vi "sub_LidarTrimPlot.vi"(0 "R_min":dbl=0.3 format="%#_13g", 1 "UDP 네트워크 연결 입력":refnum<k16>, 5 "x-":dbl=-1.0, 7 "x+":dbl=1.0, 9 "y-":dbl, 11 "y+":dbl=8.0, 12 "에러 입력(에러 없음)":errorcluster) -> (3 "UDP 네트워크 연결 출력":refnum<k16>, 4 "Point Cloud Plotting":cluster{"X":dbl, "Y":dbl}[](graph), 6 "trim XY DATA":cluster{"X":dbl, "Y":dbl}[](array[cluster]), 14 "에러 출력":errorcluster)   [LabVIEW 2020]
panel:
  in  "탭 컨트롤":enum32{"인디케이터"}(tab)
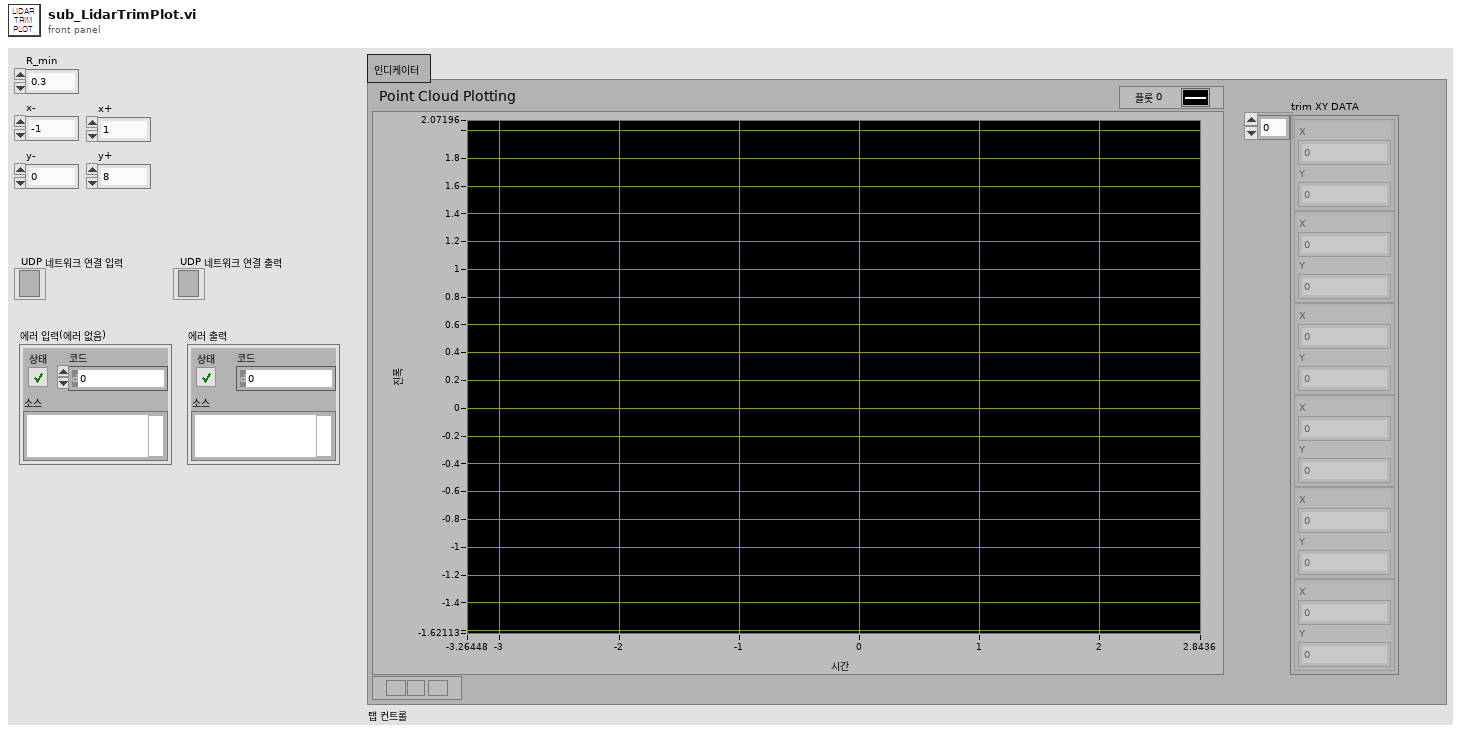
[diagram p1: front panel]
types:
  T1 = cluster{"id":i32, "azimuth (degree)":dbl, "vertical (degree)":dbl, "distance (meter)":dbl, "X":dbl, "Y":dbl, "Z":dbl}
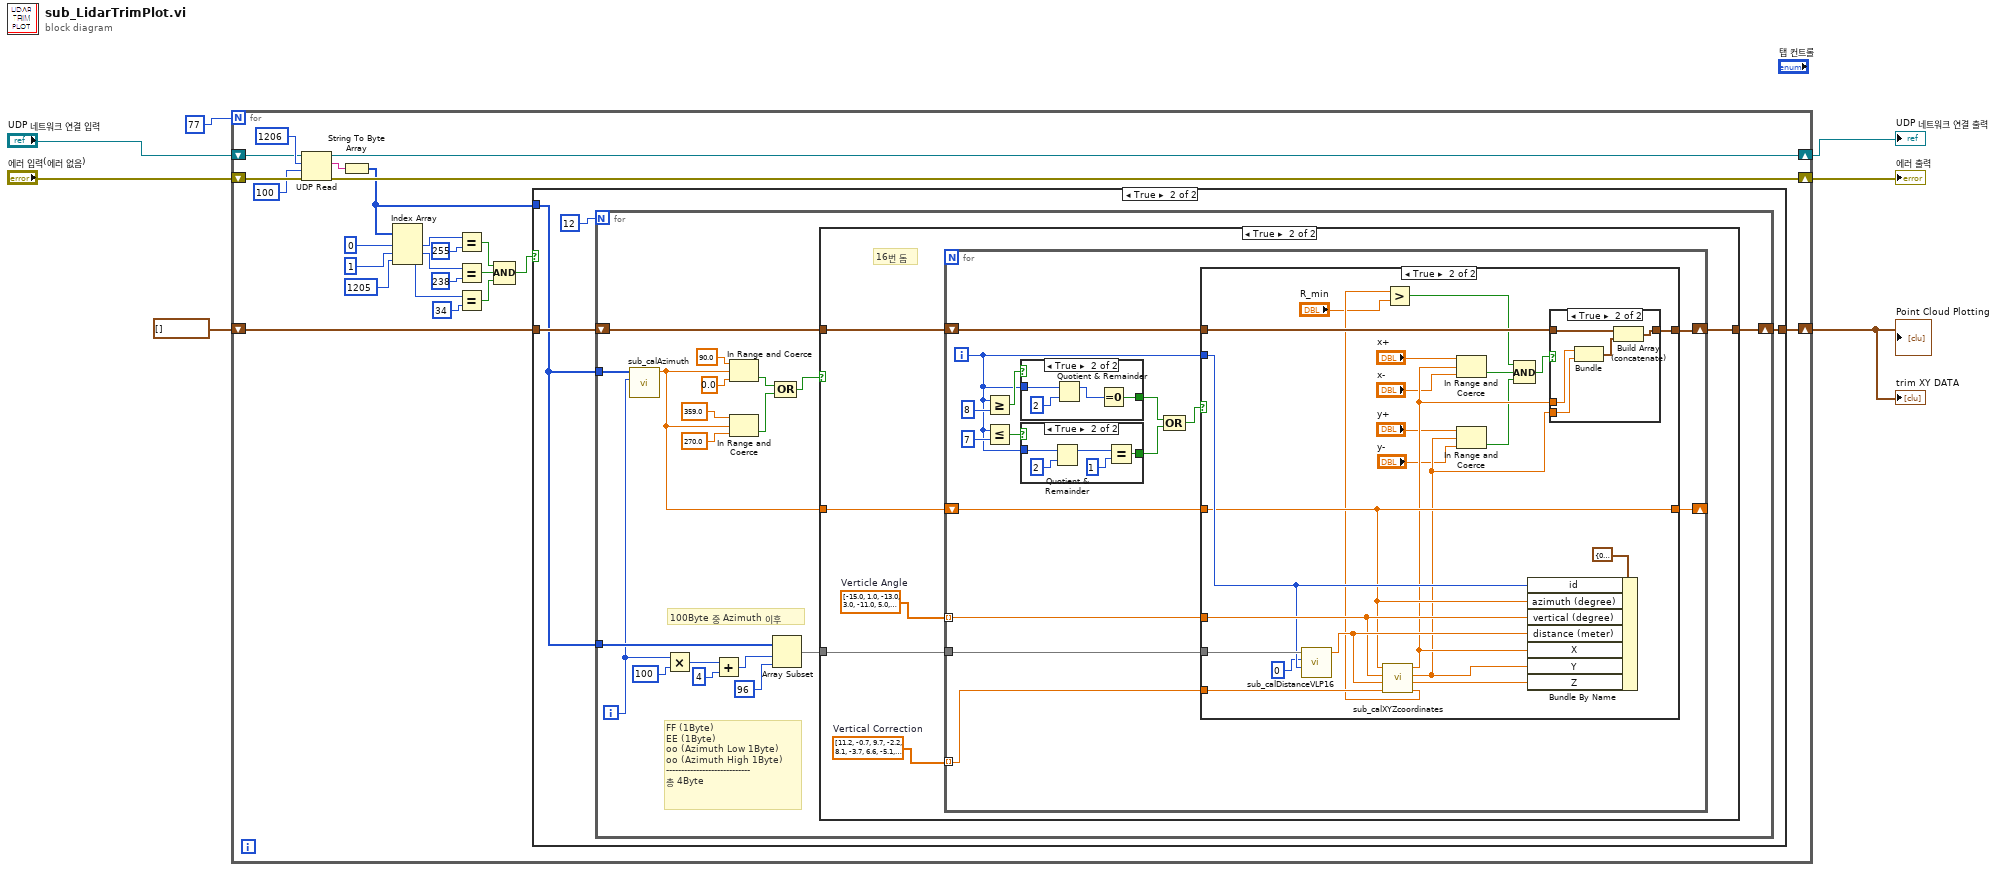
[diagram p0: block diagram]
diagram:
  n1 = for {
    N: 77 -> [_]
    shift-right: [w27] -> w3
    shift-left: "UDP 네트워크 연결 입력" -> [w29]
    shift-right: [w26] -> w4
    shift-left: "에러 입력(에러 없음)" -> [w28]
    shift-right: [w8] -> w7
    shift-left: cluster{"X":dbl, "Y":dbl}[] [] -> [w9]
    n2 = UDP Read(connection ID=w29, max size (548)=1206 ("최대 크기(548)"), timeout ms (25000)=100 ("타임아웃 ms (25000)"), 8:w28) -> (data out=w24:string, error out=w26:errorcluster, 3:w27:refnum<k16>)  [unwired: 2 out]
    n3 = String To Byte Array(string=w24) -> (unsigned byte array=w10:u8[])
    n4 = Index Array(array=w10, index #1=0 ("인덱스"), index #2=1 ("인덱스"), index #3=1205 ("인덱스")) -> (element #1=w20:u8, element #2=w18:u8, element #3=w16:u8)
    n5 = Equal?(x=w20, y=u8 255) -> (x = y?=w14:bool)
    n6 = Equal?(x=w18, y=u8 238) -> (x = y?=w13:bool)
    n7 = Equal?(x=w16, y=u8 34) -> (x = y?=w12:bool)
    n8 = Compound Arithmetic op=AND ("복합 연산")(w14, w13, w12) -> (w11:bool)
    n9 = case shown="True" w11 {
      tunnel: w10 -> [_ w32]
      tunnel: w9 -> [w31 w34]
      tunnel: [w31 w33] -> w8
      frame False {
      }
      frame True {
        n10 = for {
          N: 12 -> [_]
          tunnel: w32 -> [w49]
          shift-right: [w46] -> w33
          shift-left: w34 -> [w45]
          tunnel: w32 -> [w48]
          i -> [w47]
          # "FF (1Byte)\nEE (1Byte)\noo (Azimuth Low 1Byte)\noo (Azimuth High 1Byte)\n----------------------------\n총 4Byte"
          # "100Byte 중 Azimuth 이후"
          n11 = call "sub_calAzimuth.vi"("Index (data block)"=w47, "Byte Array"=w48) -> ("Azimuth (degree)"=w44:dbl)  [unwired: 9 in]
          n12 = Multiply(x=w47, y=100) -> (x*y=w53:i32)
          n13 = Add(x=w53, y=4) -> (x+y=w51:i32)
          n14 = In Range and Coerce(upper limit=90.0 ("상위 리미트"), x=w44, lower limit=0.0 ("하위 리미트")) -> (In Range?=w39:bool)  [unwired: 1 out]
          n15 = In Range and Coerce(upper limit=359.0 ("상위 리미트"), x=w44, lower limit=270.0 ("하위 리미트")) -> (In Range?=w38:bool)  [unwired: 1 out]
          n16 = Array Subset ("배열 잘라내기")(array=w49, index=w51, length=96 ("길이")) -> (w36:u8[])
          n17 = Compound Arithmetic op=OR ("복합 연산")(w39, w38) -> (w37:bool)
          n18 = case shown="True" w37 {
            tunnel: [w55 w61] -> w46
            tunnel: w45 -> [w55 w60]
            tunnel: w36 -> [_ w59]
            tunnel: w44 -> [_ w58]
            frame False {
            }
            frame True {
              w56 = dbl[] [11.2, -0.7, 9.7, -2.2, 8.1, -3.7, 6.6, -5.1, 5.1, -6.6, 3.7, -8.1, 2.2, -9.7, 0.7, -11.2]  # Vertical Correction
              w57 = dbl[] [-15.0, 1.0, -13.0, 3.0, -11.0, 5.0, -9.0, 7.0, -7.0, 9.0, -5.0, 11.0, -3.0, 13.0, -1.0, 15.0]  # Verticle Angle
              # "16번 돔"
              n19 = for {
                tunnel: w59 -> [w74]
                shift-right: [w73] -> w61
                shift-left: w60 -> [w76]
                tunnel: w57 -> [w75] mode=indexing
                tunnel: w56 -> [w72] mode=indexing
                shift-right: [w62] -> _
                shift-left: w58 -> [w64]
                i -> [w65]
                n20 = Greater Or Equal?(x=w65, y=8) -> (x >= y?=w71:bool)
                n21 = Less Or Equal?(x=w65, y=7) -> (x <= y?=w70:bool)
                n22 = case shown="True" w71 {
                  selector: w71 -> [w77 _]
                  tunnel: w65 -> [_ w79]
                  tunnel: [w77 w78] -> w67
                  frame False {
                  }
                  frame True {
                    n23 = Quotient & Remainder(x=w79, y=2) -> (x-y*floor(x/y)=w80:i32)  [unwired: 1 out]
                    n24 = Equal To 0?(x=w80) -> (x = 0?=w78:bool)
                  }
                }
                n25 = case shown="True" w70 {
                  selector: w70 -> [w82 _]
                  tunnel: w65 -> [_ w86]
                  tunnel: [w82 w84] -> w66
                  frame False {
                  }
                  frame True {
                    n26 = Quotient & Remainder(x=w86, y=2) -> (x-y*floor(x/y)=w85:i32)  [unwired: 1 out]
                    n27 = Equal?(x=w85, y=1) -> (x = y?=w84:bool)
                  }
                }
                n28 = Compound Arithmetic op=OR ("복합 연산")(w67, w66) -> (w63:bool)
                n29 = case shown="True" w63 {
                  tunnel: w76 -> [w89 w106]
                  tunnel: [w89 w105] -> w73
                  tunnel: w64 -> [w88 w103]
                  tunnel: w75 -> [_ w110]
                  tunnel: w65 -> [_ w108]
                  tunnel: w74 -> [_ w109]
                  tunnel: w72 -> [_ w107]
                  tunnel: [w88 w103] -> w62
                  frame False {
                  }
                  frame True {
                    n30 = call "sub_calDistanceVLP16.vi"("Index (Channel)"=w108, "Index (Firing Sequence)"=0, "Byte Array"=w109) -> ("distance (meter)"=w112:dbl)  [unwired: 8 in]
                    n31 = call "sub_calXYZcoordinates.vi"("Vertical Correction"=w107, "distance (meter)"=w112, "vertical (degree)"=w110, "azimuth (degree)"=w103) -> ("R (meter)"=w100:dbl, "Z (meter)"=w102:dbl, "Y (meter)"=w92:dbl, "X (meter)"=w101:dbl)  [unwired: 4 in]
                    n32 = Greater?(x=w100, y="R_min") -> (0:w98:bool)
                    n33 = In Range and Coerce(upper limit="x+", x=w101, lower limit="x-") -> (In Range?=w95:bool)  [unwired: 1 out]
                    n34 = In Range and Coerce(upper limit="y+", x=w92, lower limit="y-") -> (In Range?=w93:bool)  [unwired: 1 out]
                    n35 = Compound Arithmetic op=AND ("복합 연산")(w98, w95, w93) -> (w94:bool)
                    n36 = Bundle By Name(cluster=T1 {"id"=0, "azimuth (degree)"=0.0, "vertical (degree)"=0.0, "distance (meter)"=0.0, "X"=0.0, "Y"=0.0, "Z"=0.0}, "id"=w108, "azimuth (degree)"=w103, "vertical (degree)"=w110, "distance (meter)"=w112, "X"=w101, "Y"=w92, "Z"=w102) -> ()  [unwired: 1 out]
                    n37 = case shown="True" w94 {
                      tunnel: w101 -> [_ w115]
                      tunnel: w92 -> [_ w114]
                      tunnel: w106 -> [w113 w117]
                      tunnel: [w113 w116] -> w105
                      frame False {
                      }
                      frame True {
                        n38 = Bundle("X (meter)"=w115, "Y (meter)"=w114) -> (w118:cluster{"X (meter)":dbl, "Y (meter)":dbl})  [unwired: 1 in]
                        n39 = Build Array (concatenate)(w117, w118) -> (w116:cluster{"X (meter)":dbl, "Y (meter)":dbl}[])
                      }
                    }
                  }
                }
              }
            }
          }
        }
      }
    }
  }
  "Point Cloud Plotting" <- w7
  "trim XY DATA" <- w7
  "에러 출력" <- w4
  "UDP 네트워크 연결 출력" <- w3
